vi "Unit Test.vi"() -> ()   [LabVIEW 2018]
uses:
  builds/Camera.lvlibp/Custom Controls/Image Resolution.ctl
  <vilib>/vision/Image Controls.llb/IMAQ Image.ctl
  builds/Camera.lvlibp/Camera.lvclass
  <vilib>/vision/NI_Vision_Development_Module.lvlib
panel:
  in  "Image Resolution":T1=enum."1920x1200"
  out "error out":errorcluster
  in  "Sharpness":dbl
  in  "Gamma":dbl
  in  "Gain":dbl
  in  "Camera Rotation°":i16
  in  "Contrast":dbl(slide) scale=0.0..10.0
  in  "Frames Per Second":dbl
  in  "Brightness":dbl min=-10.0 max=30.0 step=1.0
  out "Image":T2(plugin-control)
  in  "stop":bool
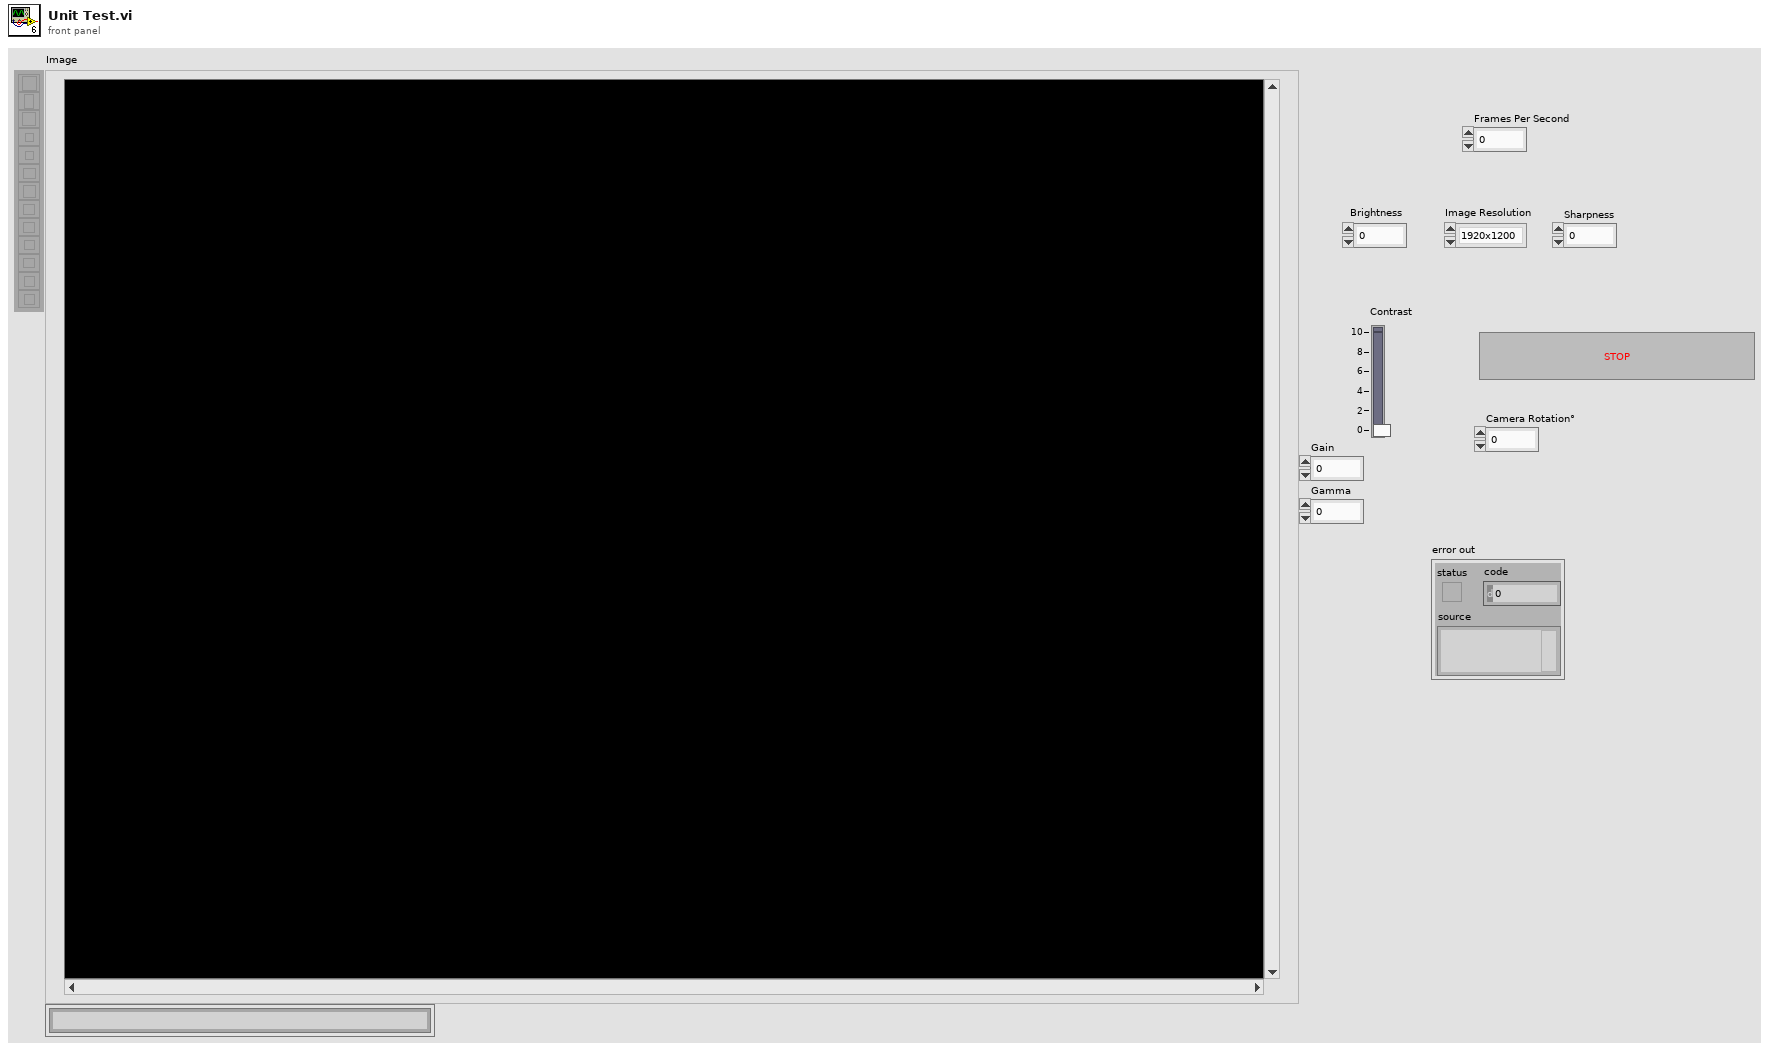
[diagram p1: front panel]
types:
  T1 = typedef "Camera.lvlibp/Camera.lvclass/Image Resolution.ctl" = enum16{"640x480", "1024x768", "1280x720", "1280x1024", "1600x1200", "1920x1080", "1920x1200"}
  T2 = typedef "IMAQ Image.ctl" = refnum<image>
  T3 = typedef "Camera.lvlibp/IMAQ Image.ctl" = refnum<image>
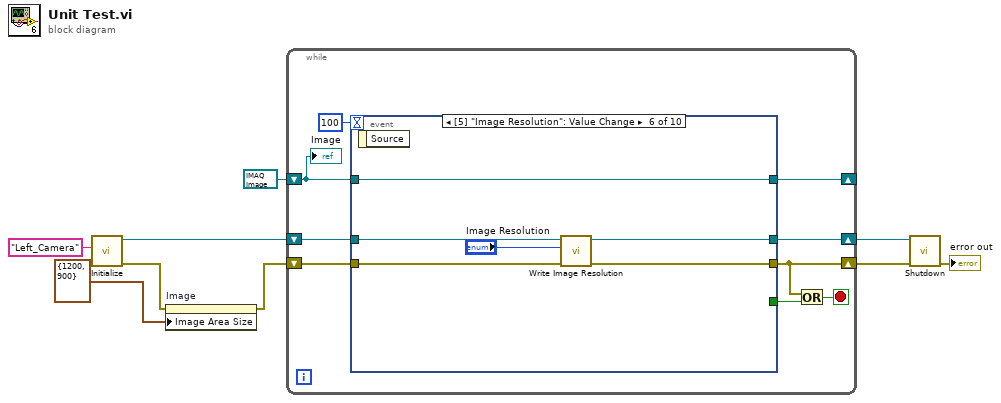
[diagram p0: block diagram]
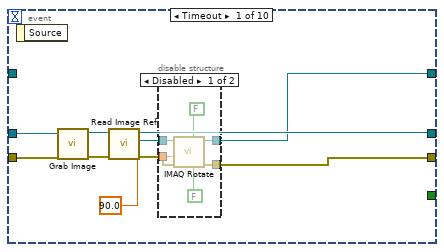
[diagram p2: hidden frame]
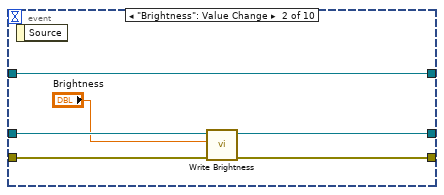
[diagram p4: hidden frame]
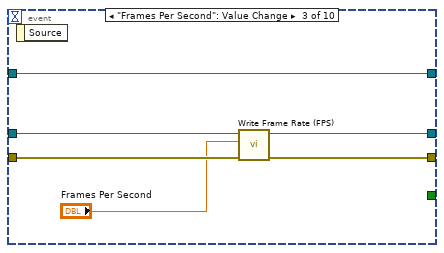
[diagram p5: hidden frame]
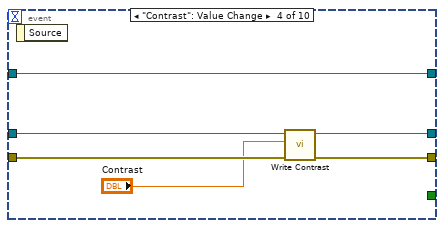
[diagram p6: hidden frame]
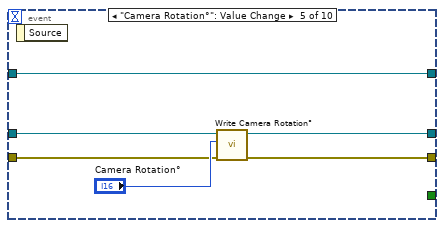
[diagram p7: hidden frame]
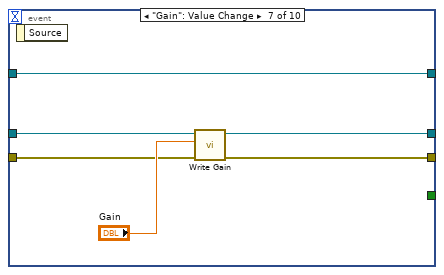
[diagram p8: hidden frame]
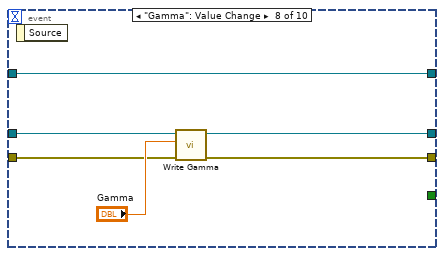
[diagram p9: hidden frame]
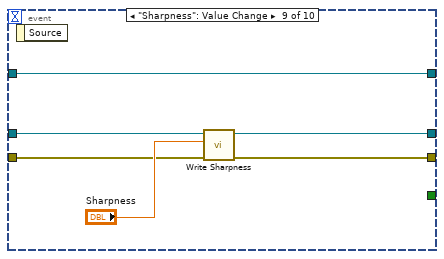
[diagram p10: hidden frame]
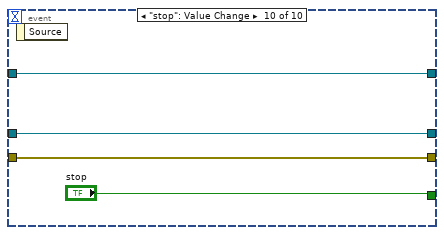
[diagram p11: hidden frame]
diagram:
  n1 = call "Initialize.vi"("Device"="Left_Camera") -> ("error out"=w5:errorcluster, "Camera out"=w9:refnum<class "Camera.lvclass">)  [unwired: 9 in]
  n2 = property on="Image" class="ImageControl"(error in=w5, "Image Area Size"=cluster{"Width":u32, "Height":u32} {"Width"=1200, "Height"=900} ("Image Area:Size:All Elements")) -> (error out=w4:errorcluster)  [unwired: 1 in, 1 out]
  n3 = while {
    shift-right: [w16] -> w8
    shift-left: w9 -> [w18]
    shift-right: [w13] -> w7
    shift-left: w4 -> [w17]
    shift-right: [w11] -> _
    shift-left: T2 refnum ("Image out") -> [w10]
    stop <- w12 stop-if-true
    n4 = event shown="[5] \"Image Resolution\": Value Change" {
      selector: _ -> [_ _ _ _ _ _ _ _ _ _]
      dyn-events: _ -> [_ _ _ _ _ _ _ _ _ _]
      timeout: 100 -> [_ _ _ _ _ _ _ _ _ _]
      tunnel: w18 -> [w27 w42 w49 w54 w59 w66 w70 w76 w82 w88]
      tunnel: w17 -> [w26 w39 w48 w53 w56 w64 w71 w77 w83 w87]
      tunnel: [w24 w41 w47 w51 w57 w65 w69 w75 w81 w88] -> w16
      tunnel: [w20 w40 w46 w52 w58 w63 w68 w74 w80 w87] -> w13
      tunnel: [_ _ _ _ _ _ _ _ _ "stop"] -> w14
      tunnel: [w19 w43 w44 w55 w61 w67 w73 w79 w85 w86] -> w11
      tunnel: w10 -> [_ w43 w44 w55 w61 w67 w73 w79 w85 w86]
      event Timeout {
        n5 = event-data() -> ()  [unwired: 1 in, 1 out]
        n6 = call-dynamic "Grab Image.vi"("error in (no error)"=w26, "Camera in"=w27) -> ("error out"=w25:errorcluster, "Camera out"=w28:refnum<class "Camera.lvclass">)  [unwired: 8 in]
        n7 = call "Read Image Ref.vi"("error in (no error)"=w25, "Camera in"=w28) -> ("error out"=w22:errorcluster, "Image"=w23:T3, "Camera out"=w24:refnum<class "Camera.lvclass">)  [unwired: 7 in]
        n8 = disable-structure shown="Disabled" {
          disable-tunnel: w23 -> [w35 w37]
          disable-tunnel: w22 -> [w34 w36]
          disable-tunnel: sgl 90.0 ("Angle (degrees)") -> [w31 _]
          disable-tunnel: [w30 w36] -> w20
          disable-tunnel: [w29 w37] -> w19
          frame Disabled {
            n9 = call "IMAQ Rotate"("Use Bilinear Interpolation"=FALSE, "Maintain Size"=FALSE, "error in (no error)"=w34, "Angle (degrees)"=w31, "Image Src"=w35) -> ("error out"=w30:errorcluster, "Image Dst Out"=w29:T2)  [unwired: 5 in]
          }
          frame Enabled {
          }
        }
      }
      event "Brightness": Value Change {
        n10 = event-data() -> ()  [unwired: 1 in, 1 out]
        n11 = call "Write Brightness.vi"("error in"=w39, "Brightness"="Brightness", "Camera in"=w42) -> ("error out"=w40:errorcluster, "Camera out"=w41:refnum<class "Camera.lvclass">)  [unwired: 7 in]
      }
      event "Frames Per Second": Value Change {
        n12 = event-data() -> ()  [unwired: 1 in, 1 out]
        n13 = call "Write Frame Rate (FPS).vi"("error in (no error)"=w48, "Frame Rate (FPS)"="Frames Per Second", "Camera in"=w49) -> ("error out"=w46:errorcluster, "Camera out"=w47:refnum<class "Camera.lvclass">)  [unwired: 7 in]
      }
      event "Contrast": Value Change {
        n14 = event-data() -> ()  [unwired: 1 in, 1 out]
        n15 = call "Write Contrast.vi"("error in"=w53, "Contrast"="Contrast", "Camera in"=w54) -> ("error out"=w52:errorcluster, "Camera out"=w51:refnum<class "Camera.lvclass">)  [unwired: 7 in]
      }
      event "Camera Rotation°": Value Change {
        n16 = event-data() -> ()  [unwired: 1 in, 1 out]
        n17 = call "Write Camera Rotation°.vi"("error in"=w56, "Camera Rotation°"="Camera Rotation°", "Camera in"=w59) -> ("error out"=w58:errorcluster, "Camera out"=w57:refnum<class "Camera.lvclass">)  [unwired: 7 in]
      }
      event Value Change {
        n18 = event-data() -> ()  [unwired: 1 in, 1 out]
        n19 = call "Write Image Resolution.vi"("error in (no error)"=w64, "Image Resolution"="Image Resolution", "Camera in"=w66) -> ("error out"=w63:errorcluster, "Camera out"=w65:refnum<class "Camera.lvclass">)  [unwired: 7 in]
      }
      event "Gain": Value Change {
        n20 = event-data() -> ()  [unwired: 1 in, 1 out]
        n21 = call "Write Gain.vi"("error in (no error)"=w71, "Gain"="Gain", "Camera in"=w70) -> ("error out"=w68:errorcluster, "Camera out"=w69:refnum<class "Camera.lvclass">)  [unwired: 7 in]
      }
      event "Gamma": Value Change {
        n22 = event-data() -> ()  [unwired: 1 in, 1 out]
        n23 = call "Write Gamma.vi"("error in (no error)"=w77, "Gamma"="Gamma", "Camera in"=w76) -> ("error out"=w74:errorcluster, "Camera out"=w75:refnum<class "Camera.lvclass">)  [unwired: 7 in]
      }
      event "Sharpness": Value Change {
        n24 = event-data() -> ()  [unwired: 1 in, 1 out]
        n25 = call "Write Sharpness.vi"("error in"=w83, "Sharpness"="Sharpness", "Camera in"=w82) -> ("error out"=w80:errorcluster, "Camera out"=w81:refnum<class "Camera.lvclass">)  [unwired: 7 in]
      }
      event "stop": Value Change {
        n26 = event-data() -> ()  [unwired: 1 in, 1 out]
      }
    }
    n27 = Or(x=w13, y=w14) -> (x .or. y?=w12:bool)
    "Image" <- w10
  }
  n28 = call "Shutdown.vi"("error in"=w7, "Camera in"=w8) -> ("error out"=→"error out":errorcluster)  [unwired: 8 in, 1 out]
